vi "Hello.vi"() -> ()   [LabVIEW 2017]
panel:
  in  "Boolean":bool
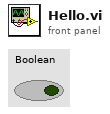
[diagram p1: front panel]
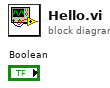
[diagram p0: block diagram]
diagram:
